vi "Extrapolate Path Ending.vi"(10 "Lookahead":dbl, 11 "Path in":T1[](array[typedef])) -> (2 "End Point":i32, 3 "Path out":T1[](array[typedef]))   [LabVIEW 2017, in "Pure Pursuit.lvlib"]
uses:
  Typedef/Path Point.ctl
  Pure Pursuit.lvlib
  <vilib>/ptbypt/NI_PtbyPt.lvlib
panel:
  out "XY Graph":cluster{dbl[], dbl[]}[](graph)
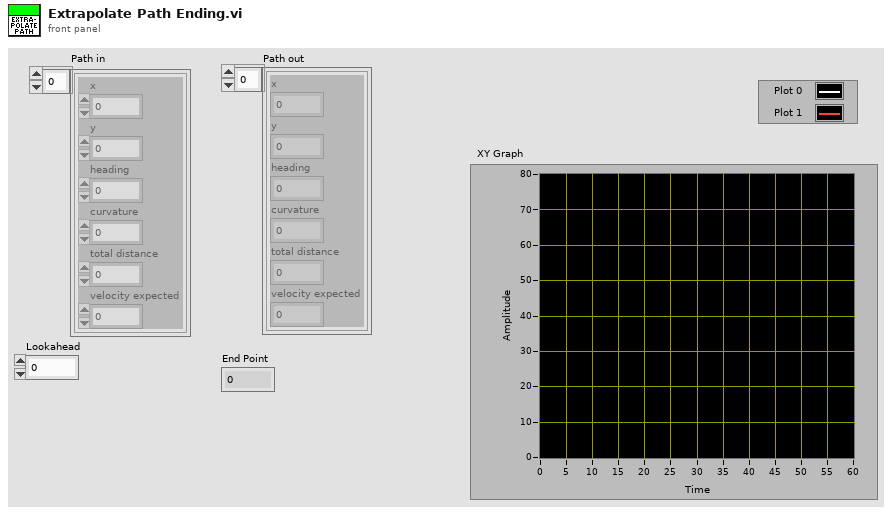
[diagram p1: front panel]
types:
  T1 = typedef "Pure Pursuit.lvlib/Path Point.ctl" = cluster{"x":dbl, "y":dbl, "heading":dbl, "curvature":dbl, "total distance":dbl, "velocity expected":dbl}
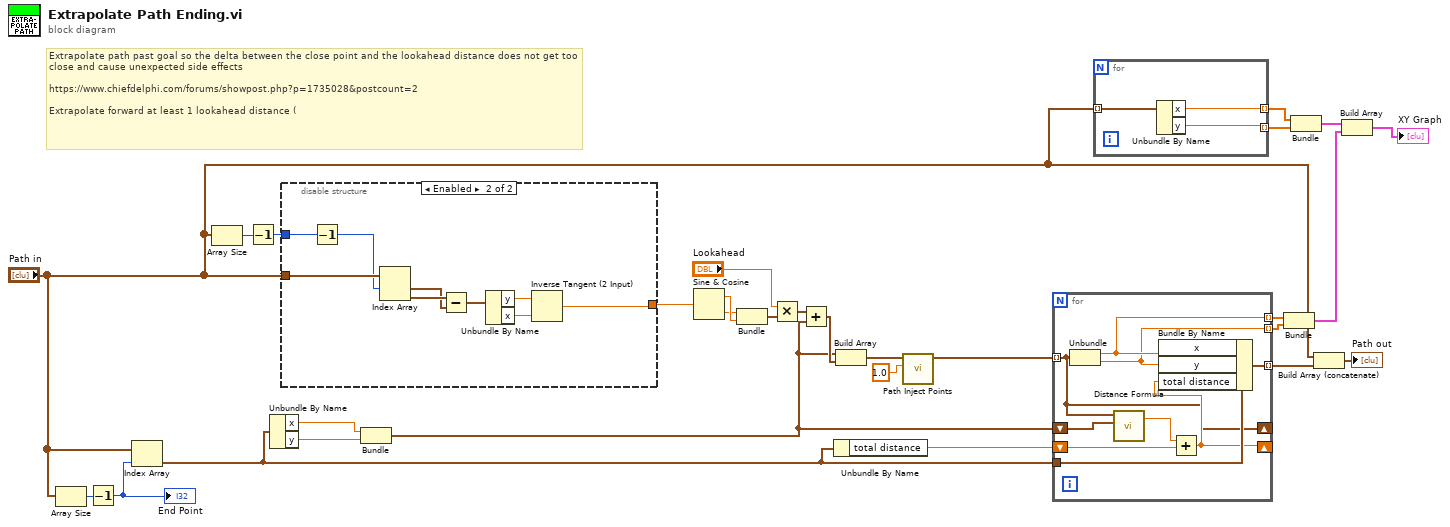
[diagram p0: block diagram]
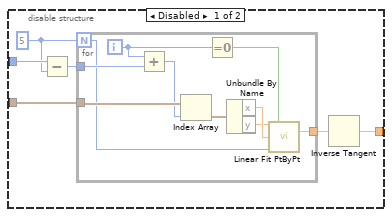
[diagram p2: hidden frame]
diagram:
  # "Extrapolate path past goal so the delta between the close point and the lookahead distance does not get too close and cause unexpected side effects\n\nhttps://www.chiefdelphi.com/forums/showpost.php?p=1735028&postcount=2\n\nExtrapolate forward at least 1 lookahead distance ("
  n1 = Array Size(array="Path in") -> (size(s)=w28:i32)
  n2 = Decrement(x=w28) -> (x-1=w29:i32)
  "End Point" <- w29
  n3 = Index Array(array="Path in", index=w29) -> (element=w5:T1)
  n4 = Array Size(array="Path in") -> (size(s)=w27:i32)
  n5 = Decrement(x=w27) -> (x-1=w26:i32)
  n6 = Unbundle By Name(w5) -> ("x"=w23:dbl, "y"=w22:dbl)
  n7 = disable-structure shown="Enabled" {
    disable-tunnel: w26 -> [w35 w53]
    disable-tunnel: "Path in" -> [w32 w54]
    disable-tunnel: [w30 w49] -> w1
    frame Disabled {
      w33 = 5
      n8 = Subtract(x=w35, y=w33) -> (x-y=w34:i32)
      n9 = for {
        N: w33 -> [w37]
        tunnel: w32 -> [w44]
        tunnel: w34 -> [w45]
        tunnel: [w36] -> w31
        i -> [w39]
        n10 = Add(x=w39, y=w45) -> (x+y=w43:i32)
        n11 = Index Array(array=w44, index=w43) -> (element=w42:T1)
        n12 = Equal To 0?(x=w39) -> (x = 0?=w38:bool)
        n13 = Unbundle By Name(w42) -> ("x"=w41:dbl, "y"=w40:dbl)
        n14 = call <vilib>:"Linear Fit PtByPt.vi"("y"=w40, "initialize"=w38, "x"=w41, "sample length"=w37) -> ("slope"=w36:dbl)  [unwired: 7 in, 4 out]
      }
      n15 = Inverse Tangent(1:w31) -> (0:w30:dbl)
    }
    frame Enabled {
      n16 = Decrement(x=w53) -> (x-1=w52:i32)
      n17 = Index Array(array=w54, index #1=w52) -> (element #1=w50:T1, element #2=w51:T1)  [unwired: 1 in]
      n18 = Subtract(x=w51, y=w50) -> (x-y=w48:T1)
      n19 = Unbundle By Name(w48) -> ("y"=w47:dbl, "x"=w46:dbl)
      n20 = Inverse Tangent (2 Input)(1:w46, 2:w47) -> (0:w49:dbl)
    }
  }
  n21 = Bundle("x"=w23, "y"=w22) -> (w3:cluster{"x":dbl, "y":dbl})  [unwired: 1 in]
  n22 = Sine & Cosine(0:w1) -> (1:w25:dbl, 2:w24:dbl)
  n23 = Bundle(w24, w25) -> (w21:cluster{dbl, dbl})  [unwired: 1 in]
  n24 = Multiply(x="Lookahead", y=w21) -> (x*y=w17:cluster{dbl, dbl})
  n25 = Add(x=w17, y=w3) -> (x+y=w19:cluster{dbl, dbl})
  n26 = Unbundle By Name(w5) -> ("total distance"=w4:dbl)
  n27 = Build Array(w3, w19) -> (w18:cluster{"x":dbl, "y":dbl}[])
  n28 = call "Path Inject Points.vi"("Distance"=1.0, "Path"=w18) -> ("Path out"=w2:cluster{dbl, dbl}[])  [unwired: 9 in]
  n29 = for {
    tunnel: w2 -> [w55] mode=indexing
    tunnel: w5 -> [w63]
    tunnel: [w62] -> w14 mode=indexing
    tunnel: [w61] -> w10 mode=indexing
    tunnel: [w60] -> w9 mode=indexing
    shift-right: [w55] -> _
    shift-left: w3 -> [w59]
    shift-right: [w56] -> _
    shift-left: w4 -> [w57]
    n30 = Unbundle(w55) -> (w61:dbl, w60:dbl)
    n31 = call "Distance Formula.vi"("Point2"=w59, "Point1"=w55) -> ("Distance"=w58:dbl)  [unwired: 3 in]
    n32 = Add(x=w58, y=w57) -> (x+y=w56:dbl)
    n33 = Bundle By Name(cluster=w63, "x"=w61, "y"=w60, "total distance"=w56) -> (w62:T1)
  }
  n34 = for {
    tunnel: "Path in" -> [w66] mode=indexing
    tunnel: [w65] -> w11 mode=indexing
    tunnel: [w64] -> w12 mode=indexing
    n35 = Unbundle By Name(w66) -> ("x"=w65:dbl, "y"=w64:dbl)
  }
  n36 = Bundle(w10, w9) -> (w8:cluster{dbl[], dbl[]})  [unwired: 1 in]
  n37 = Bundle(w11, w12) -> (w7:cluster{dbl[], dbl[]})  [unwired: 1 in]
  n38 = Build Array (concatenate)("Path in", w14) -> (→"Path out":T1[])
  n39 = Build Array(w7, w8) -> (→"XY Graph":cluster{dbl[], dbl[]}[])
